vi "Config目录.vi"() -> ()   [LabVIEW 2013]
panel:
  in  "ConfigĿ¼":path=path "D:/研究生/课程/油动机项目/12-交付/油动机性能测试仪/油动机分析测试软件2017-12-20/Config"
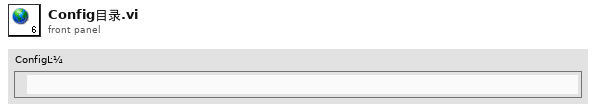
[diagram p1: front panel]
diagram:
